vi "myRIO_BRig_Host_v0,35__PortC.vi"() -> ()   [LabVIEW 2014]
panel:
  out "graph_ai1":dbl(graph)
  out "RunTime_seconds":u16
  out "RunTime_minutes":u16
  out "BlockL_T2R_cur":u16 caption="Trials2Reward"
  out "BlockL_BTPR_cur":u16 caption="BadTrialsPostReward"
  out "BlockL_T2R_avg":dbl caption="Trials2Reward" format="%#_3g"
  out "BlockL_BTPR_avg":dbl caption="BadTrialsPostReward" format="%#_3g"
  out "BlockR_T2R_cur":u16 caption="Trials2Reward"
  out "BlockR_BTPR_cur":u16 caption="BadTrialsPostReward"
  out "BlockR_T2R_avg":dbl caption="Trials2Reward" format="%#_3g"
  out "BlockR_BTPR_avg":dbl caption="BadTrialsPostReward" format="%#_3g"
  out "error_LoadPrevSettings":errorcluster caption="error out"
  in  "LoadPrevSettings":bool
  out "graph_ai0":dbl(graph)
  in  "maxTrialsDisplayed":i32 caption="Number of Trials Displayed\n( 0 = all trials )"
  out "error_TCP":errorcluster
  in  "stop":bool
  in  "colorIn_timeout":u32(colorbox)=7468543 caption="Choice Timeout"
  in  "colorIn_wrong/cue":u32(colorbox)=16728618 caption="Wrong Choice"
  in  "colorIn_reward":u32(colorbox)=5898088 caption="Reward"
  in  "colorIn_unknown":u32(colorbox)=16449331 caption="Unknown Trial Status"
  out "dataOut_plot":cluster{i32[], i32[]}[](graph)
  out "iTrial":i32
  out "iBlock":i32
  # "Current Block Stats"
  # "Trials 2 Reward\n\nBad Trials Post Reward"
  # "Left         Right"
  # "Run Time\n   minutes    seconds"
  # "Average Block Stats"
  # "Trials 2 Reward\n\nBad Trials Post Reward"
  # "Left         Right"
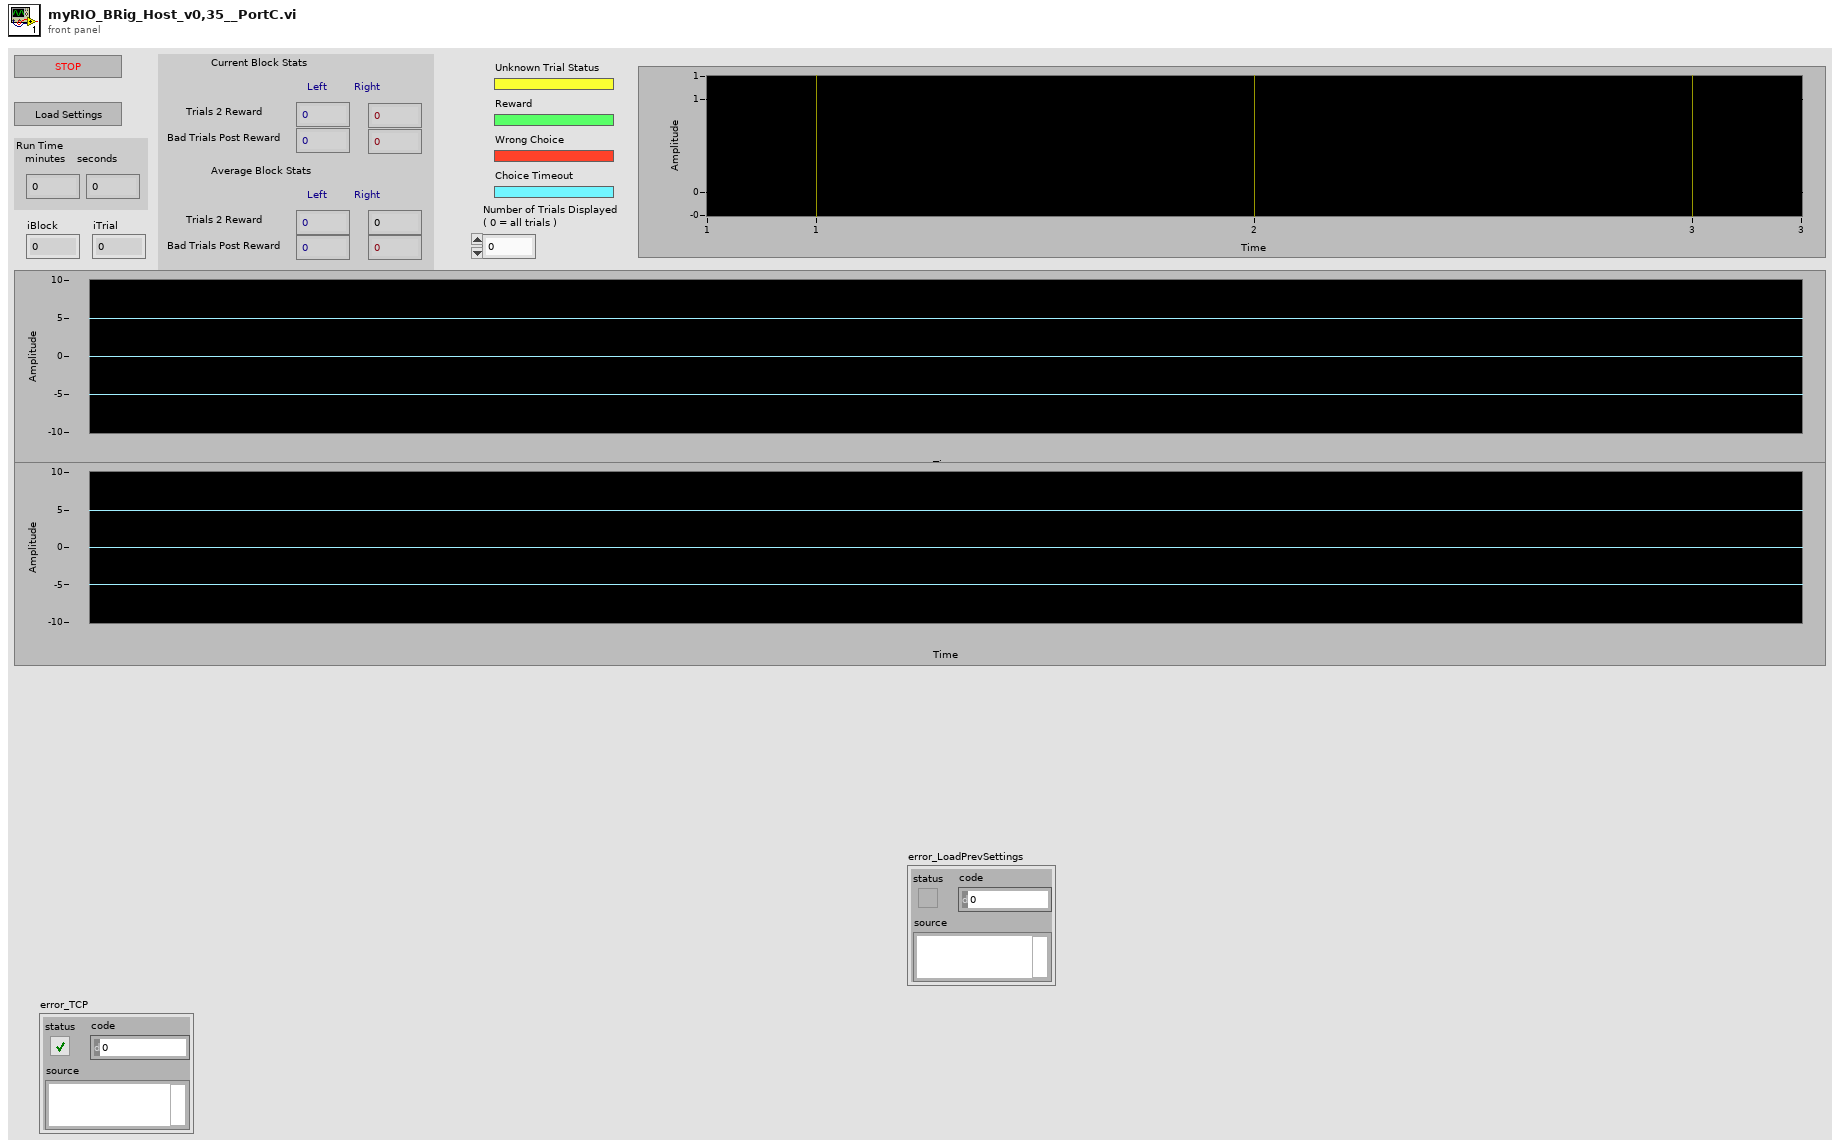
[diagram p1: front panel]
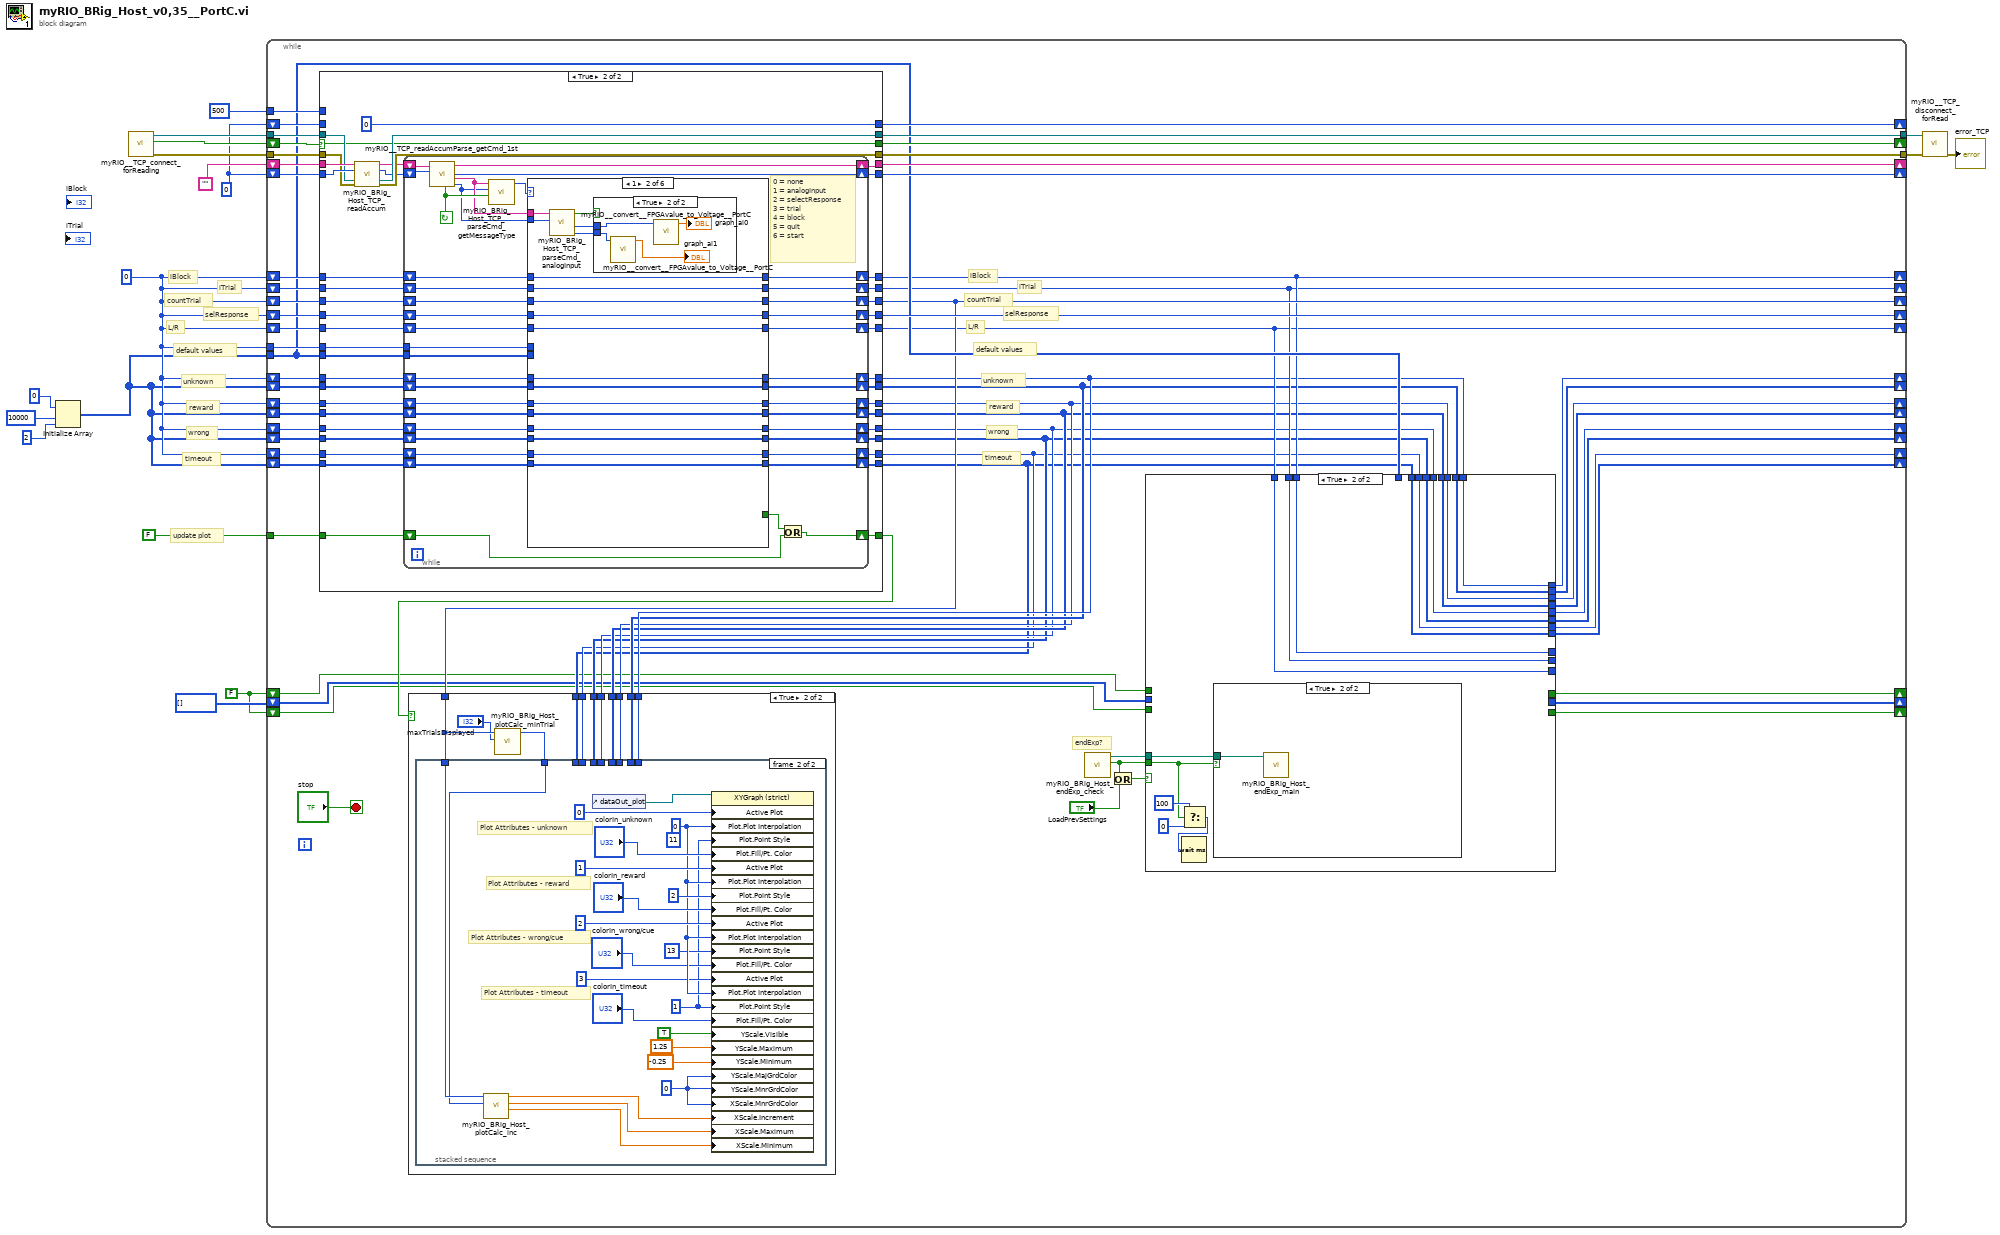
[diagram p0: block diagram]
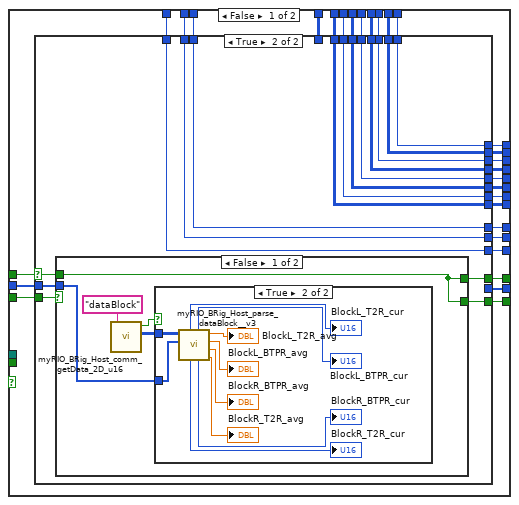
[diagram p2: hidden frame]
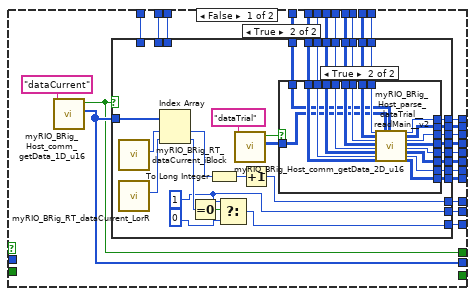
[diagram p3: hidden frame]
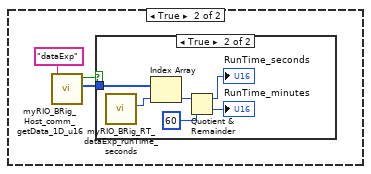
[diagram p7: hidden frame]
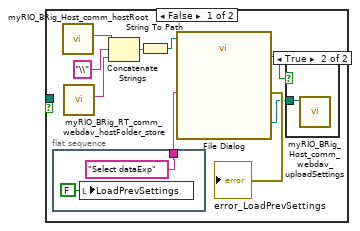
[diagram p9: hidden frame]
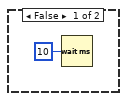
[diagram p11: hidden frame]
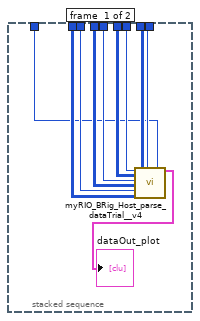
[diagram p12: hidden frame]
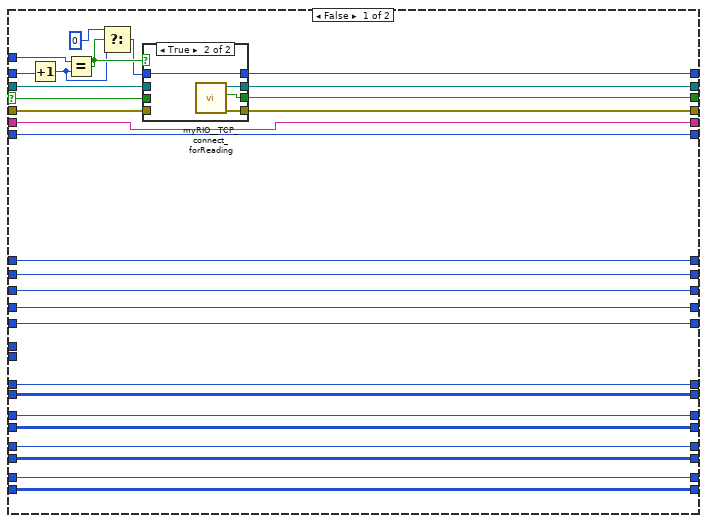
[diagram p13: hidden frame]
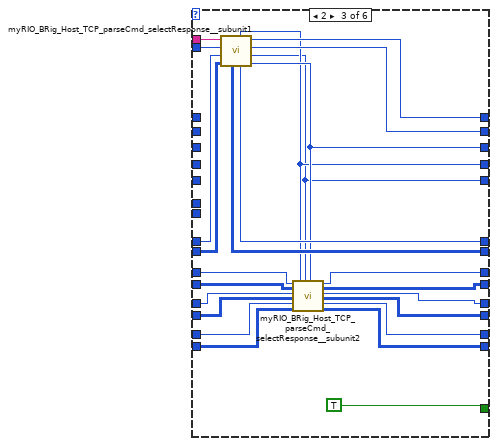
[diagram p17: hidden frame]
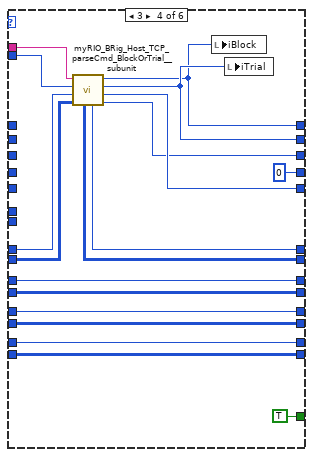
[diagram p18: hidden frame]
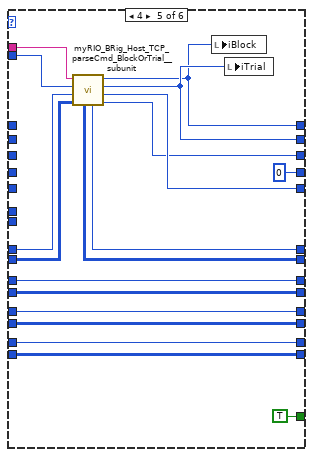
[diagram p19: hidden frame]
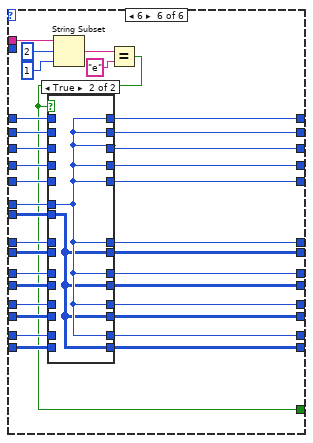
[diagram p20: hidden frame]
diagram:
  w1 = FALSE ("output_I_data")
  w4 = 0
  w13 = 0
  # "default values"
  # "update plot"
  # "timeout"
  # "wrong"
  # "reward"
  # "unknown"
  # "L/R"
  # "selResponse"
  # "countTrial"
  # "iBlock"
  # "iTrial"
  n1 = Initialize Array(0 ("element"), 10000 ("dimension size"), 2 ("dimension size")) -> (w3:i32[][])
  n2 = call "myRIO__TCP_connect_forReading.vi"() -> ("output_error"=w15:errorcluster, "output_connected"=w16:bool, "output_hTCP"=w17:refnum<k5>)  [unwired: 9 in]
  n3 = while {
    tunnel: w17 -> [w78]
    tunnel: w15 -> [w76]
    shift-right: [w69] -> _
    shift-left: w13 -> [w74]
    shift-right: [w70] -> _
    shift-left: "" -> [w75]
    shift-right: [w71] -> _
    shift-left: w16 -> [w77]
    shift-right: [w72] -> _
    shift-left: w13 -> [w79]
    tunnel: 500 ("y") -> [w73]
    shift-right: [w42] -> _
    shift-left: w4 -> [w68]
    shift-right: [w41] -> _
    shift-left: w4 -> [w67]
    shift-right: [w43] -> _
    shift-left: w4 -> [w66]
    shift-right: [w54] -> _
    shift-left: w4 -> [w65]
    shift-right: [w40] -> _
    shift-left: w4 -> [w64]
    shift-right: [w31] -> _
    shift-left: w4 -> [w63]
    shift-right: [w30] -> _
    shift-left: w3 -> [w62]
    shift-right: [w29] -> _
    shift-left: w4 -> [w61]
    shift-right: [w28] -> _
    shift-left: w3 -> [w60]
    shift-right: [w27] -> _
    shift-left: w4 -> [w59]
    shift-right: [w26] -> _
    shift-left: w3 -> [w58]
    shift-right: [w25] -> _
    shift-left: w4 -> [w57]
    shift-right: [w24] -> _
    shift-left: w3 -> [w56]
    tunnel: [w52] -> w7
    tunnel: [w51] -> w6
    tunnel: FALSE -> [w55]
    tunnel: w4 -> [w49]
    tunnel: w3 -> [w44]
    shift-right: [w23] -> _
    shift-left: u16[] [] ("output_data_1D") -> [w20]
    shift-right: [w22] -> _
    shift-left: w1 -> [w21]
    shift-right: [w18] -> _
    shift-left: w1 -> [w19]
    stop <- "stop" stop-if-true
    # "default values"
    # "timeout"
    # "wrong"
    # "reward"
    # "unknown"
    # "L/R"
    # "selResponse"
    # "countTrial"
    # "iBlock"
    # "iTrial"
    # "endExp?"
    n4 = case shown="True" w77 {
      selector: w77 -> [w338 w387]
      tunnel: w75 -> [w332 w393]
      tunnel: w74 -> [w333 w392]
      tunnel: [w332 w383] -> w70
      tunnel: [w333 w382] -> w69
      tunnel: w78 -> [w339 w391]
      tunnel: [w342 w390] -> w52
      tunnel: w76 -> [w337 w389]
      tunnel: [w341 w388] -> w51
      tunnel: [w340 w387] -> w71
      tunnel: w79 -> [w343 _]
      tunnel: [w331 0] -> w72
      tunnel: w73 -> [w330 _]
      tunnel: w68 -> [w329 w381]
      tunnel: w67 -> [w328 w380]
      tunnel: w66 -> [w327 w379]
      tunnel: w65 -> [w326 w378]
      tunnel: w64 -> [w325 w377]
      tunnel: w63 -> [w324 w376]
      tunnel: w62 -> [w323 w375]
      tunnel: w61 -> [w322 w374]
      tunnel: w60 -> [w321 w373]
      tunnel: w59 -> [w320 w372]
      tunnel: w58 -> [w319 w371]
      tunnel: w57 -> [w318 w370]
      tunnel: w56 -> [w317 w369]
      tunnel: w55 -> [_ w368]
      tunnel: [_ w367] -> w53
      tunnel: [w329 w366] -> w42
      tunnel: [w328 w365] -> w41
      tunnel: [w327 w364] -> w43
      tunnel: [w326 w363] -> w54
      tunnel: [w325 w362] -> w40
      tunnel: [w324 w361] -> w39
      tunnel: [w323 w360] -> w38
      tunnel: [w322 w359] -> w37
      tunnel: [w321 w358] -> w36
      tunnel: [w320 w357] -> w35
      tunnel: [w319 w356] -> w34
      tunnel: [w318 w355] -> w33
      tunnel: [w317 w354] -> w32
      tunnel: w49 -> [_ w353]
      tunnel: w44 -> [_ w352]
      frame False {
        n5 = Increment(x=w343) -> (x+1=w316:i32)
        n6 = Equal?(x=w330, y=w316) -> (x = y?=w336:bool)
        n7 = Select(t=0, s=w336, f=w316) -> (s? t:f=w334:i32)
        n8 = case shown="True" w336 {
          tunnel: w334 -> [w344 w348]
          tunnel: [w347 w351] -> w342
          tunnel: [w345 w350] -> w341
          tunnel: [w346 w349] -> w340
          tunnel: w339 -> [w347 _]
          tunnel: w338 -> [w346 _]
          tunnel: w337 -> [w345 _]
          tunnel: [w344 w348] -> w331
          frame False {
          }
          frame True {
            n9 = call "myRIO__TCP_connect_forReading.vi"() -> ("output_error"=w350:errorcluster, "output_connected"=w349:bool, "output_hTCP"=w351:refnum<k5>)  [unwired: 9 in]
          }
        }
      }
      frame True {
        n10 = call "myRIO_BRig_Host_TCP_readAccum.vi"("input_strAccum"=w393, "input_count"=w392, "input_handle_TCP"=w391, "input_error"=w389) -> ("output_strAccum"=w385:string, "output_count"=w384:i32, "output_handle_TCP"=w390:refnum<k5>, "output_error"=w388:errorcluster)  [unwired: 8 in]
        n11 = while {
          shift-right: [w430] -> w383
          shift-left: w385 -> [w432]
          shift-right: [w429] -> w382
          shift-left: w384 -> [w431]
          shift-right: [w421] -> w366
          shift-left: w381 -> [w424]
          shift-right: [w420] -> w365
          shift-left: w380 -> [w423]
          shift-right: [w419] -> w364
          shift-left: w379 -> [w422]
          shift-right: [w417] -> w363
          shift-left: w378 -> [w418]
          shift-right: [w415] -> w362
          shift-left: w377 -> [w416]
          shift-right: [w413] -> w361
          shift-left: w376 -> [w414]
          shift-right: [w411] -> w360
          shift-left: w375 -> [w412]
          shift-right: [w404] -> w359
          shift-left: w374 -> [w410]
          shift-right: [w403] -> w358
          shift-left: w373 -> [w409]
          shift-right: [w402] -> w357
          shift-left: w372 -> [w408]
          shift-right: [w401] -> w356
          shift-left: w371 -> [w407]
          shift-right: [w399] -> w354
          shift-left: w369 -> [w405]
          shift-right: [w400] -> w355
          shift-left: w370 -> [w406]
          shift-right: [w397] -> w367
          shift-left: w368 -> [w394]
          tunnel: w353 -> [w396]
          tunnel: w352 -> [w395]
          stop <- w428 continue-if-true
          # "0 = none\n1 = analogInput\n2 = selectResponse\n3 = trial\n4 = block\n5 = quit\n6 = start"
          n12 = call "myRIO__TCP_readAccumParse_getCmd_1st.vi"("input_count"=w431, "input_strAccum"=w432) -> ("output_countCmd"=w426:i32, "output_strCmd"=w427:string, "output_count"=w429:i32, "output_strAccum"=w430:string, "output_haveCmd"=w428:bool)  [unwired: 5 in]
          n13 = call "myRIO_BRig_Host_TCP_parseCmd_getMessageType.vi"("input_haveCmd"=w428, "input_countCmd"=w426, "input_strCmd"=w427) -> ("output_messageType"=w425:u8)  [unwired: 8 in]
          n14 = case shown="1" w425 {
            tunnel: w427 -> [_ w450 w491 w508 w526 w561]
            tunnel: w426 -> [_ w449 w490 w507 w525 _]
            tunnel: w424 -> [w445 w463 _ _ _ w556]
            tunnel: w423 -> [w444 w462 _ _ _ w554]
            tunnel: w422 -> [w443 w461 _ _ _ w553]
            tunnel: [w445 w463 w485 w493 w511 w555] -> w421
            tunnel: [w444 w462 w484 w494 w512 w550] -> w420
            tunnel: [w443 w461 w483 w501 w519 w549] -> w419
            tunnel: w418 -> [w442 w460 _ _ _ w552]
            tunnel: [w442 w460 w482 0 ("output_iTrial_num") 0 ("output_iTrial_num") w548] -> w417
            tunnel: w416 -> [w441 w459 _ _ _ w551]
            tunnel: [w441 w459 w481 w502 w520 w547] -> w415
            tunnel: w414 -> [w440 w458 w489 w506 w524 w546]
            tunnel: [w440 w458 w487 w504 w522 w538] -> w413
            tunnel: w412 -> [w439 w457 w488 w505 w523 w545]
            tunnel: [w439 w457 w486 w503 w521 w537] -> w411
            tunnel: w410 -> [w438 w456 w480 w500 w518 w544]
            tunnel: w409 -> [w437 w455 w479 w499 w517 w543]
            tunnel: w408 -> [w436 w454 w478 w498 w516 w542]
            tunnel: w407 -> [w435 w453 w477 w497 w515 w541]
            tunnel: w406 -> [w434 w452 w476 w496 w514 w540]
            tunnel: w405 -> [w433 w451 w475 w495 w513 w539]
            tunnel: [w438 w456 w474 w500 w518 w536] -> w404
            tunnel: [w437 w455 w473 w499 w517 w535] -> w403
            tunnel: [w436 w454 w472 w498 w516 w534] -> w402
            tunnel: [w435 w453 w471 w497 w515 w533] -> w401
            tunnel: [w434 w452 w470 w496 w514 w532] -> w400
            tunnel: [w433 w451 w469 w495 w513 w531] -> w399
            tunnel: [_ _ TRUE TRUE TRUE w528] -> w398
            tunnel: w396 -> [_ _ _ _ _ w530]
            tunnel: w395 -> [_ _ _ _ _ w529]
            frame 0, Default {
            }
            frame 1 {
              n15 = call "myRIO_BRig_Host_TCP_parseCmd_analogInput.vi"("input_countCmd"=w449, "input_strCmd"=w450) -> ("output_ai1"=w446:i32, "output_ai0"=w447:i32, "output_haveAnalogInput"=w448:bool)  [unwired: 7 in]
              n16 = case shown="True" w448 {
                tunnel: w447 -> [_ w467]
                tunnel: w446 -> [_ w465]
                frame False {
                }
                frame True {
                  n17 = call "myRIO__convert__FPGAvalue_to_Voltage__PortC.vi"("input_FPGAvalue_PortC"=w465) -> ("output_voltage"=→"graph_ai1":dbl)  [unwired: 10 in]
                  n18 = call "myRIO__convert__FPGAvalue_to_Voltage__PortC.vi"("input_FPGAvalue_PortC"=w467) -> ("output_voltage"=→"graph_ai0":dbl)  [unwired: 10 in]
                }
              }
            }
            frame 2 {
              n19 = call "myRIO_BRig_Host_TCP_parseCmd_selectResponse__subunit1.vi"("input_arrayUnknown"=w488, "input_idxUnknown"=w489, "input_countCmd"=w490, "input_strCmd"=w491) -> ("output_countTrial"=w483:i32, "output_L/R"=w481:i32, "output_iTrial"=w484:i32, "output_iBlock"=w485:i32, "output_idxUnknown"=w487:i32, "output_response"=w482:i32, "output_arrayUnknown"=w486:i32[][])  [unwired: 1 in]
              n20 = call "myRIO_BRig_Host_TCP_parseCmd_selectResponse__subunit2.vi"("input_idxReward"=w480, "input_arrayReward"=w479, "input_idxWrong"=w478, "input_arrayWrong"=w477, "input_idxTimeout"=w476, "input_arrayTimeout"=w475, "input_response"=w482, "input_L/R"=w481, "input_countTrial"=w483) -> ("output_idxReward"=w474:i32, "output_arrayReward"=w473:i32[][], "output_idxWrong"=w472:i32, "output_arrayWrong"=w471:i32[][], "output_idxTimeout"=w470:i32, "output_arrayTimeout"=w469:i32[][])  [unwired: 5 in]
            }
            frame 3 {
              n21 = call "myRIO_BRig_Host_TCP_parseCmd_BlockOrTrial__subunit.vi"("input_arrayUnknown"=w505, "input_idxUnknown"=w506, "input_countCmd"=w507, "input_strCmd"=w508) -> ("output_countTrial"=w501:i32, "output_L/R"=w502:i32, "output_iTrial"=w494:i32, "output_iBlock"=w493:i32, "output_idxUnknown"=w504:i32, "output_arrayUnknown"=w503:i32[][])  [unwired: 2 in]
              n22 = local write "iBlock"(w493) -> ()
              n23 = local write "iTrial"(w494) -> ()
            }
            frame 4 {
              n24 = call "myRIO_BRig_Host_TCP_parseCmd_BlockOrTrial__subunit.vi"("input_arrayUnknown"=w523, "input_idxUnknown"=w524, "input_countCmd"=w525, "input_strCmd"=w526) -> ("output_countTrial"=w519:i32, "output_L/R"=w520:i32, "output_iTrial"=w512:i32, "output_iBlock"=w511:i32, "output_idxUnknown"=w522:i32, "output_arrayUnknown"=w521:i32[][])  [unwired: 2 in]
              n25 = local write "iBlock"(w511) -> ()
              n26 = local write "iTrial"(w512) -> ()
            }
            frame 6 {
              n27 = String Subset(string=w561, offset (0)=2, length (rest)=1 ("length (rest)")) -> (substring=w558:string)
              n28 = Equal?(x=w558, y="e") -> (x = y?=w528:bool)
              n29 = case shown="True" w528 {
                tunnel: w556 -> [w574 _]
                tunnel: [w574 w576] -> w555
                tunnel: w554 -> [w573 _]
                tunnel: w553 -> [w572 _]
                tunnel: w552 -> [w571 _]
                tunnel: w551 -> [w570 _]
                tunnel: [w573 w576] -> w550
                tunnel: [w572 w576] -> w549
                tunnel: [w571 w576] -> w548
                tunnel: [w570 w576] -> w547
                tunnel: w546 -> [w569 _]
                tunnel: w545 -> [w568 _]
                tunnel: w544 -> [w567 _]
                tunnel: w543 -> [w566 _]
                tunnel: w542 -> [w565 _]
                tunnel: w541 -> [w564 _]
                tunnel: w540 -> [w563 _]
                tunnel: w539 -> [w562 _]
                tunnel: [w569 w576] -> w538
                tunnel: [w568 w575] -> w537
                tunnel: [w567 w576] -> w536
                tunnel: [w566 w575] -> w535
                tunnel: [w565 w576] -> w534
                tunnel: [w564 w575] -> w533
                tunnel: [w563 w576] -> w532
                tunnel: [w562 w575] -> w531
                tunnel: w530 -> [_ w576]
                tunnel: w529 -> [_ w575]
                frame False {
                }
                frame True {
                }
              }
            }
          }
          n30 = Or(x=w398, y=w394) -> (x .or. y?=w397:bool)
        }
      }
    }
    n31 = case shown="True" w53 {
      tunnel: w32 -> [_ w283]
      tunnel: w33 -> [_ w282]
      tunnel: w34 -> [_ w281]
      tunnel: w35 -> [_ w280]
      tunnel: w36 -> [_ w279]
      tunnel: w37 -> [_ w278]
      tunnel: w38 -> [_ w277]
      tunnel: w39 -> [_ w276]
      tunnel: w43 -> [_ w275]
      frame False {
        n32 = Wait (ms)(milliseconds to wait=u32 10) -> ()  [unwired: 1 out]
      }
      frame True {
        n33 = call "myRIO_BRig_Host_plotCalc_minTrial.vi"("input_maxTrialsDisplayed"="maxTrialsDisplayed", "input_countTrial"=w275) -> ("output_minTrial"=w273:i32)  [unwired: 9 in]
        n34 = stacked-sequence {
          tunnel: w283 -> [w293 _]
          tunnel: w282 -> [w292 _]
          tunnel: w281 -> [w291 _]
          tunnel: w280 -> [w290 _]
          tunnel: w279 -> [w289 _]
          tunnel: w278 -> [w288 _]
          tunnel: w277 -> [w287 _]
          tunnel: w276 -> [w286 _]
          tunnel: w273 -> [w284 w297]
          tunnel: w275 -> [_ w298]
          frame #0 {
            n35 = call "myRIO_BRig_Host_parse_dataTrial__v4.vi"("input_idxReward"=w288, "input_arrayReward"=w289, "input_idxWrong"=w290, "input_arrayWrong"=w291, "input_idxTimeout"=w292, "input_arrayTimeout"=w293, "input_arrayUnknown"=w287, "input_idxUnknown"=w286, "input_minTrial"=w284) -> ("output_plotData"=→"dataOut_plot":cluster{i32[], i32[]}[])  [unwired: 10 in]
          }
          frame #1 {
            w300 = u32 0 ("Y Scale.Grid Colors:Major Color")
            w299 = u8 1 ("Plot.Point Style")
            (unwired) u8 11 ("Plot.Point Style")
            w309 = u8 0 ("Plot.Plot Interpolation")
            # "Plot Attributes - timeout"
            # "Plot Attributes - wrong/cue"
            # "Plot Attributes - reward"
            # "Plot Attributes - unknown"
            n36 = call "myRIO_BRig_Host_plotCalc_inc.vi"("input_minTrial"=w297, "input_countTrial"=w298) -> ("output_min"=w294:dbl, "output_max"=w295:dbl, "output_inc"=w296:dbl)  [unwired: 7 in]
            n37 = control-ref of="dataOut_plot"() -> (w304:refnum<vi>)
            n38 = property on="Property Node" class="XYGraph (strict)"(reference=w304, "Active Plot"=u32 0, "Plot.Plot Interpolation"=w309, "Plot.Point Style"=w299, "Plot.Fill/Pt. Color"="colorIn_unknown", "Active Plot"=u32 1, "Plot.Plot Interpolation"=w309, "Plot.Point Style"=u8 2, "Plot.Fill/Pt. Color"="colorIn_reward", "Active Plot"=u32 2, "Plot.Plot Interpolation"=w309, "Plot.Point Style"=u8 13, "Plot.Fill/Pt. Color"="colorIn_wrong/cue", "Active Plot"=u32 3, "Plot.Plot Interpolation"=w309, "Plot.Point Style"=w299, "Plot.Fill/Pt. Color"="colorIn_timeout", "YScale.Visible"=TRUE ("Y Scale.Visible"), "YScale.Maximum"=1.25 ("Y Scale.Range:Maximum"), "YScale.Minimum"=-0.25 ("Y Scale.Range:Minimum"), "YScale.MajGrdColor"=w300, "YScale.MnrGrdColor"=w300, "XScale.MnrGrdColor"=w300, "XScale.Increment"=w296, "XScale.Maximum"=w295, "XScale.Minimum"=w294) -> ()  [unwired: 1 in, 2 out]
          }
        }
      }
    }
    n39 = call "myRIO_BRig_Host_endExp_check.vi"() -> ("output_IendExp"=w46:bool, "output_filePath_expExp"=w45:path)  [unwired: 10 in]
    n40 = Or(x=w46, y="LoadPrevSettings") -> (x .or. y?=w47:bool)
    n41 = case shown="True" w47 {
      tunnel: w46 -> [_ w255]
      tunnel: w45 -> [_ w254]
      tunnel: [w108 w253] -> w31
      tunnel: [w107 w252] -> w30
      tunnel: [w106 w251] -> w29
      tunnel: [w105 w250] -> w28
      tunnel: [w104 w249] -> w27
      tunnel: [w103 w248] -> w26
      tunnel: [w102 w247] -> w25
      tunnel: [w101 w246] -> w24
      tunnel: w39 -> [w100 w253]
      tunnel: w38 -> [w99 w252]
      tunnel: w37 -> [w98 w251]
      tunnel: w36 -> [w97 w250]
      tunnel: w35 -> [w96 w249]
      tunnel: w34 -> [w95 w248]
      tunnel: w33 -> [w94 w247]
      tunnel: w32 -> [w93 w246]
      tunnel: w44 -> [w92 _]
      tunnel: [w91 w243] -> _
      tunnel: [w90 w244] -> _
      tunnel: [w89 w245] -> _
      tunnel: w42 -> [w88 w245]
      tunnel: w41 -> [w87 w244]
      tunnel: w40 -> [w86 w243]
      tunnel: [w85 _] -> w23
      tunnel: [w84 _] -> w22
      tunnel: w21 -> [w83 _]
      tunnel: w20 -> [w82 _]
      tunnel: w19 -> [w81 _]
      tunnel: [w80 _] -> w18
      frame False {
        n42 = case shown="True" w83 {
          selector: w83 -> [_ w204]
          tunnel: [w133 w218] -> w108
          tunnel: [w132 w217] -> w107
          tunnel: [w131 w216] -> w106
          tunnel: [w130 w215] -> w105
          tunnel: [w129 w214] -> w104
          tunnel: [w128 w213] -> w103
          tunnel: [w127 w212] -> w102
          tunnel: [w126 w211] -> w101
          tunnel: w100 -> [w125 w218]
          tunnel: w99 -> [w124 w217]
          tunnel: w98 -> [w123 w216]
          tunnel: w97 -> [w122 w215]
          tunnel: w96 -> [w121 w214]
          tunnel: w95 -> [w120 w213]
          tunnel: w94 -> [w119 w212]
          tunnel: w93 -> [w118 w211]
          tunnel: w92 -> [w117 _]
          tunnel: [w116 w208] -> w91
          tunnel: [w115 w209] -> w90
          tunnel: [w114 w210] -> w89
          tunnel: w88 -> [w113 w210]
          tunnel: w87 -> [w112 w209]
          tunnel: w86 -> [w111 w208]
          tunnel: [w110 _] -> w85
          tunnel: [w109 w205] -> w84
          tunnel: w82 -> [_ w207]
          tunnel: w81 -> [_ w206]
          tunnel: [_ w203] -> w80
          frame False {
            n43 = call "myRIO_BRig_Host_comm_getData_1D_u16.vi"("input_fileName"="dataCurrent") -> ("output_data_1D"=w110:u16[], "output_I_data"=w109:bool)  [unwired: 9 in]
            n44 = case shown="True" w109 {
              tunnel: w110 -> [_ w176]
              tunnel: [w145 w171] -> w133
              tunnel: [w144 w170] -> w132
              tunnel: [w143 w169] -> w131
              tunnel: [w142 w168] -> w130
              tunnel: [w141 w167] -> w129
              tunnel: [w140 w166] -> w128
              tunnel: [w139 w165] -> w127
              tunnel: [w138 w164] -> w126
              tunnel: w125 -> [w145 w163]
              tunnel: w124 -> [w144 w162]
              tunnel: w123 -> [w143 w161]
              tunnel: w122 -> [w142 w160]
              tunnel: w121 -> [w141 w159]
              tunnel: w120 -> [w140 w158]
              tunnel: w119 -> [w139 w157]
              tunnel: w118 -> [w138 w156]
              tunnel: w117 -> [_ w155]
              tunnel: [w135 w151] -> w116
              tunnel: [w136 w150] -> w115
              tunnel: [w137 w146] -> w114
              tunnel: w113 -> [w137 _]
              tunnel: w112 -> [w136 _]
              tunnel: w111 -> [w135 _]
              frame False {
              }
              frame True {
                w150 = 1
                n45 = call "myRIO_BRig_RT_dataCurrent_iBlock.vi"() -> ("output_iBlock"=w149:i32)  [unwired: 11 in]
                n46 = call "myRIO_BRig_RT_dataCurrent_LorR.vi"() -> ("output_LorR"=w172:i32)  [unwired: 11 in]
                n47 = Index Array(array=w176, index #1=w149, index #2=w172) -> (element #1=w148:u16, element #2=w154:u16)
                n48 = Equal To 0?(x=w154) -> (x = 0?=w153:bool)
                n49 = To Long Integer(number=w148) -> (32bit integer=w147:i32)
                n50 = Select(t=w150, s=w153, f=0) -> (s? t:f=w151:i32)
                n51 = call "myRIO_BRig_Host_comm_getData_2D_u16.vi"("input_fileName"="dataTrial") -> ("output_data_2D"=w173:u16[][], "output_I_data"=w174:bool)  [unwired: 9 in]
                n52 = Increment(x=w147) -> (x+1=w146:i32)
                n53 = case shown="True" w174 {
                  tunnel: w173 -> [_ w194]
                  tunnel: [w182 w190] -> w169
                  tunnel: [w181 w189] -> w168
                  tunnel: [w183 w191] -> w170
                  tunnel: [w184 w192] -> w171
                  tunnel: [w180 w188] -> w167
                  tunnel: [w179 w187] -> w166
                  tunnel: [w178 w186] -> w165
                  tunnel: [w177 w185] -> w164
                  tunnel: w155 -> [_ w193]
                  tunnel: w163 -> [w184 w202]
                  tunnel: w162 -> [w183 w201]
                  tunnel: w161 -> [w182 w200]
                  tunnel: w160 -> [w181 w199]
                  tunnel: w159 -> [w180 w198]
                  tunnel: w158 -> [w179 w197]
                  tunnel: w157 -> [w178 w196]
                  tunnel: w156 -> [w177 w195]
                  frame False {
                  }
                  frame True {
                    n54 = call "myRIO_BRig_Host_parse_dataTrial__readMain__v2.vi"("input_idxUnknown"=w202, "input_arrayUnknown"=w201, "input_idxReward"=w200, "input_arrayReward"=w199, "input_idxWrong"=w198, "input_arrayWrong"=w197, "input_idxTimeout"=w196, "input_arrayTimeout"=w195, "arrayIn_dataTrial"=w194, "arrayIn_empty"=w193) -> ("output_idxUnknown"=w192:i32, "output_arrayUnknown"=w191:i32[][], "output_idxReward"=w190:i32, "output_arrayReward"=w189:i32[][], "output_idxWrong"=w188:i32, "output_arrayWrong"=w187:i32[][], "output_idxTimeout"=w186:i32, "output_arrayTimeout"=w185:i32[][])  [unwired: 10 in]
                  }
                }
              }
            }
          }
          frame True {
            n55 = case shown="False" w206 {
              tunnel: w207 -> [w220 _]
              tunnel: [w219 _] -> w205
              tunnel: w204 -> [w219 _]
              tunnel: [w219 _] -> w203
              frame False {
                n56 = call "myRIO_BRig_Host_comm_getData_2D_u16.vi"("input_fileName"="dataBlock") -> ("output_data_2D"=w221:u16[][], "output_I_data"=w222:bool)  [unwired: 9 in]
                n57 = case shown="True" w222 {
                  tunnel: w221 -> [_ w225]
                  tunnel: w220 -> [_ w224]
                  frame False {
                  }
                  frame True {
                    n58 = call "myRIO_BRig_Host_parse_dataBlock__v3.vi"("input_dataCurrent"=w224, "input_dataBlock"=w225) -> ("BlockR_T2R_avg"=→"BlockR_T2R_avg":dbl, "BlockR_BTPR_avg"=→"BlockR_BTPR_avg":dbl, "BlockL_BTPR_avg"=→"BlockL_BTPR_avg":dbl, "BlockL_T2R_avg"=→"BlockL_T2R_avg":dbl, "BlockR_BTPR_cur"=→"BlockR_BTPR_cur":u16, "BlockL_BTPR_cur"=→"BlockL_BTPR_cur":u16, "BlockR_T2R_cur"=→"BlockR_T2R_cur":u16, "BlockL_T2R_cur"=→"BlockL_T2R_cur":u16)  [unwired: 2 in]
                  }
                }
              }
              frame True {
                n59 = call "myRIO_BRig_Host_comm_getData_1D_u16.vi"("input_fileName"="dataExp") -> ("output_data_1D"=w236:u16[], "output_I_data"=w235:bool)  [unwired: 9 in]
                n60 = case shown="True" w235 {
                  tunnel: w236 -> [_ w242]
                  frame False {
                  }
                  frame True {
                    n61 = call "myRIO_BRig_RT_dataExp_runTime_seconds.vi"() -> ("output_RunTime_minutes"=w241:i32)  [unwired: 11 in]
                    n62 = Index Array(array=w242, index=w241) -> (element=w240:u16)
                    n63 = Quotient & Remainder(x=w240, y=u16 60) -> (x-y*floor(x/y)=→"RunTime_seconds":u16, floor(x/y)=→"RunTime_minutes":u16)
                  }
                }
              }
            }
          }
        }
      }
      frame True {
        n64 = Select(t=u32 100 ("milliseconds to wait"), s=w255, f=u32 0 ("milliseconds to wait")) -> (s? t:f=w257:u32)
        n65 = Wait (ms)(milliseconds to wait=w257) -> ()  [unwired: 1 out]
        n66 = case shown="True" w255 {
          tunnel: w254 -> [_ w271]
          frame False {
            n67 = flat-sequence {
              tunnel: ["Select dataExp" ("prompt")] -> w262
              frame #0 {
                n68 = local write "LoadPrevSettings"(FALSE ("LoadPrevSettings")) -> ()
              }
            }
            n69 = call "myRIO_BRig_Host_comm_hostRoot.vi"() -> ("output_hostRoot"=w264:string)  [unwired: 11 in]
            n70 = call "myRIO_BRig_RT_comm_webdav_hostFolder_store.vi"() -> ("output_HostFolder"=w266:string)  [unwired: 11 in]
            n71 = Concatenate Strings(w264, "\\" ("string"), w266) -> (w267:string)
            n72 = String To Path(string=w267) -> (path=w263:path)
            n73 = call "File Dialog"("start path"=w263, "prompt"=w262) -> ("selected path"=w259:path, "exists"=w260:bool, "error out"=→"error_LoadPrevSettings":errorcluster)  [unwired: 10 in, 1 out]
            n74 = case shown="True" w260 {
              tunnel: w259 -> [_ w268]
              frame False {
              }
              frame True {
                n75 = call "myRIO_BRig_Host_comm_webdav_uploadSettings.vi"("input_filePath"=w268) -> ()  [unwired: 11 in]
              }
            }
          }
          frame True {
            n76 = call "myRIO_BRig_Host_endExp_main.vi"("input_filePath"=w271) -> ()  [unwired: 11 in]
          }
        }
      }
    }
  }
  n77 = call "myRIO__TCP_disconnect_forRead.vi"("input_error"=w6, "input_hTCP"=w7) -> ("output_error"=→"error_TCP":errorcluster)  [unwired: 9 in]
